vi "trythree.vi"() -> ()   [LabVIEW 2019]
uses:
  libtrythree.dll
panel:
  in  "Kd":dbl
  out "return type":dbl
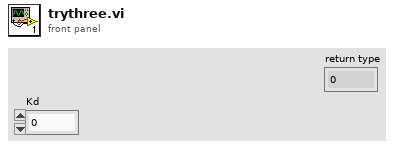
[diagram p1: front panel]
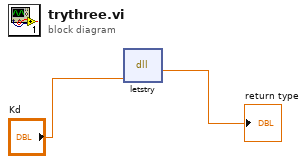
[diagram p0: block diagram]
diagram:
  n1 = dll-call lib="libtrythree.*" fn="letstry"("arg1"="Kd") -> ("return type"=→"return type":dbl)  [unwired: 4 in, 2 out]
